vi "Parse Buffer.vi"(8 "error in (no error)":errorcluster, 11 "Buffer":u8[](array[numeric]) format="%02x") -> (0 "error out":errorcluster, 3 "Raw Fields":T1[](array[typedef]))   [LabVIEW 2020, in "Protobuf RAW.lvlib"]
uses:
  Protobuf RAW.lvlib
  Wire Chunk.ctl
  Type Serializer/Wire Type.ctl
  Wire Type Group/Wire Type Group.lvclass
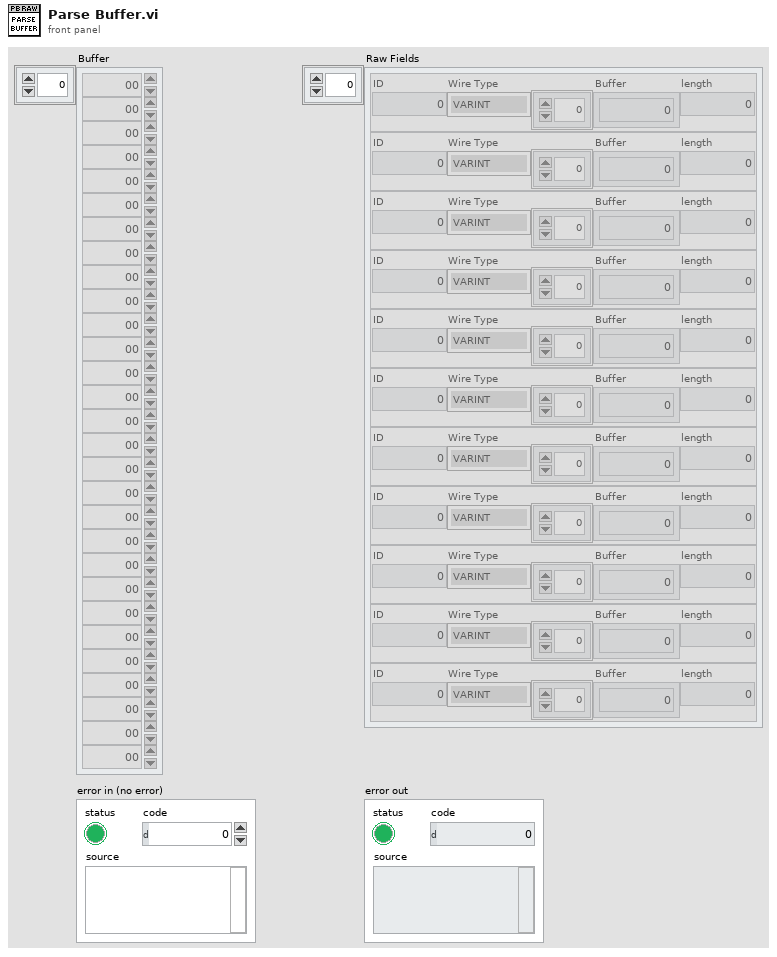
[diagram p1: front panel]
types:
  T1 = typedef "Protobuf RAW.lvlib/Wire Chunk.ctl" = cluster{"ID":u32, "Wire Type":T2, "Buffer":u8[], "length":i32}
  T2 = typedef "Protobuf RAW.lvlib/Wire Type Group.lvclass/Wire Type.ctl" = enum16{"VARINT", "I64", "LEN", "SGROUP", "EGROUP", "I32"}
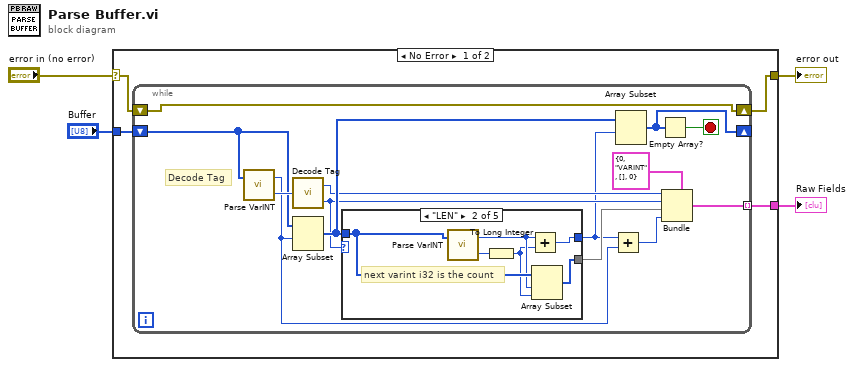
[diagram p0: block diagram]
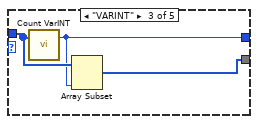
[diagram p3: hidden frame]
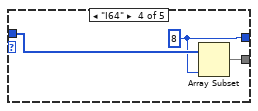
[diagram p4: hidden frame]
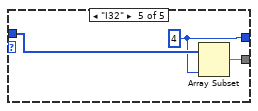
[diagram p5: hidden frame]
diagram:
  n1 = case shown="No Error" "error in (no error)" {
    selector: "error in (no error)" -> [w6 w38]
    tunnel: [w8 w38] -> w4
    tunnel: [w7 _] -> w3
    tunnel: "Buffer" -> [w5 _]
    frame No Error {
      n2 = while {
        shift-right: [w19] -> _
        shift-left: w5 -> [w21]
        shift-right: [w13] -> w8
        shift-left: w6 -> [w13]
        tunnel: [w15] -> w7 mode=indexing
        stop <- w18 stop-if-true
        # "Decode Tag"
        n3 = call "Parse VarINT.vi"("Buffer"=w21) -> ("Numeric"=w22:u64, "Bytes"=w10:i32)  [unwired: 1 in]
        n4 = call "Decode Tag.vi"("Tag"=w22) -> ("ID"=w14:u32, "Wire Type"=w17:T2)
        n5 = Array Subset(array=w21, index=w10) -> (w20:u8[])  [unwired: 1 in]
        n6 = case shown="\"LEN\"" w17 {
          tunnel: w20 -> [_ w27 w31 w34 w37]
          tunnel: [_ w26 w30 w33 w36] -> w12
          tunnel: [_ w23 w29 w32 w35] -> w9
          frame Default {
          }
          frame "LEN" {
            # "next varint i32 is the count"
            n7 = call "Parse VarINT.vi"("Buffer"=w27) -> ("Numeric"=w28:u64, "Bytes"=w25:i32)  [unwired: 1 in]
            n8 = To Long Integer(number=w28) -> (32bit integer=w24:i32)
            n9 = Add(x=w25, y=w24) -> (x+y=w23:i32)
            n10 = Array Subset(array=w27, index=w25, length=w24) -> (w26:u8[])
          }
          frame "VARINT" {
            n11 = call "Count VarINT.vi"("Buffer"=w31) -> ("Bytes"=w29:i32)  [unwired: 2 in]
            n12 = Array Subset(array=w31, length=w29) -> (w30:u8[])  [unwired: 1 in]
          }
          frame "I64" {
            w32 = 8 ("length")
            n13 = Array Subset(array=w34, length=w32) -> (w33:u8[])  [unwired: 1 in]
          }
          frame "I32" {
            w35 = 4 ("length")
            n14 = Array Subset(array=w37, length=w35) -> (w36:u8[])  [unwired: 1 in]
          }
        }
        n15 = Add(x=w9, y=w10) -> (x+y=w11:i32)
        n16 = Array Subset(array=w20, index=w9) -> (w19:u8[])  [unwired: 1 in]
        n17 = Empty Array?(array=w19) -> (empty?=w18:bool)
        n18 = Bundle(cluster=T1 {"ID"=0, "Wire Type"=enum."VARINT", "Buffer"=[], "length"=0} ("output cluster"), "ID"=w14, "Wire Type"=w17, "Buffer"=w12, "length"=w11) -> (w15:T1)
      }
    }
    frame Error {
    }
  }
  "error out" <- w4
  "Raw Fields" <- w3
